vi "Test Assetion Results Records Assertion Type.vi"(8 "error in (no error)":errorcluster, 11 "Test Case In":refnum<class "Result Collector Tests.lvclass">) -> (0 "error out":errorcluster, 3 "Test Case Out":refnum<class "Result Collector Tests.lvclass">)   [LabVIEW 2020, in "Result Collector Tests.lvclass"]
uses:
  Result Collector Tests.lvclass
  C:/Program Files (x86)/National Instruments/LabVIEW 2020/vi.lib/Astemes/LUnit/Test Case.lvclass
  source/Framework/Result Collector/Result Collector.lvclass
  source/Rewrite Project/Result/Result.ctl
  source/Rewrite Project/Result/Status.ctl
  source/Rewrite Project/Result/Type.ctl
  source/Framework/Result Types/Assertion Result/Public/TypeDefs/Assertion Type.ctl
  source/Framework/Result Collector/Result Collector.lvclass/Result Collector.ctl
  <vilib>/Astemes/LUnit/Test Case.lvclass/Test Case.ctl
  7d523b10-b8d1-4baa-9334-5865d033fd32.vi
  source/Framework/Result Collector/Public/API/Collect Method Results.vi
  <vilib>/AdvancedString/Delimited String to 1D String Array.vi
  <vilib>/AdvancedString/1D String Array to Delimited String.vi
  source/Framework/Result Collector/Public/API/Collect Case Result.vi
  source/Framework/Result Collector/Public/API/Collect Suite Result.vi
  <vilib>/Astemes/LUnit/Palette/Pass.vi
  <vilib>/Astemes/LUnit/Palette/Fail.vi
  <vilib>/Astemes/LUnit/Compare Variants.vi
  <vilib>/Astemes/LUnit/Describe Comparison.vi
  <vilib>/Astemes/LUnit/Set Assertion Type.vi
  <vilib>/Astemes/LUnit/Add test result.vi
  <vilib>/Astemes/LUnit/Variant to string.vi
  <vilib>/Astemes/LUnit/LUnit Record Assertion Result.vi
  <vilib>/Astemes/LUnit/LUnit Aggregate Assertion Results.vi
  <vilib>/Astemes/LUnit/Method Result/LUnit Merge Status.vi
  <vilib>/Astemes/LUnit/LUnit Concatenate result strings.vi
  <vilib>/Utility/Data Type/Get Type Information.vi
  <vilib>/Utility/LVClass/Get LV Class Name.vi
  source/Rewrite Project/Result/Result.lvlib
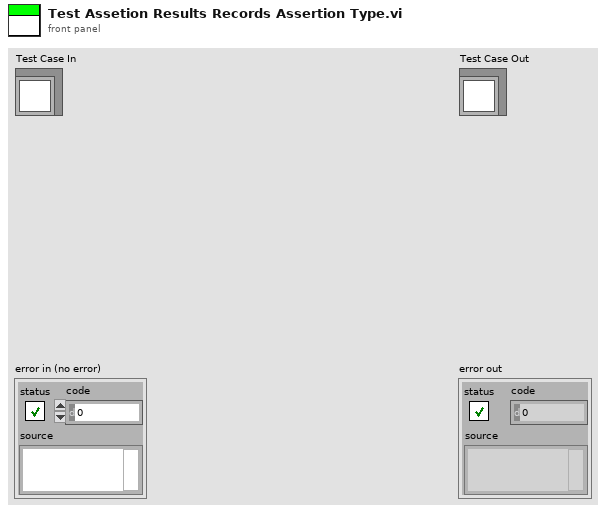
[diagram p1: front panel]
types:
  T1 = typedef "Result.lvlib/Assertion Type.ctl" = enum16{"None", "Pass", "Fail", "Skip", "Pass if Equal", "Fail if Equal", "Pass if Error", "Fail if Error", "Pass if", "Fail if"}
  T2 = typedef "Result.lvlib/Result.ctl" = cluster{"Name":string, "Message":string, "Description":string, "Status":T3, "Result Type":T4, "Execution Time":dbl}
  T3 = typedef "Result.lvlib/Status.ctl" = enum16{"", "Passed", "Failed", "Error", "Skipped", "Setup Error", "Broken", "Teardown Error"}
  T4 = typedef "Result.lvlib/Type.ctl" = enum16{"Method", "Case", "Suite", "Pass", "Fail", "Skip", "Pass if", "Fail if", "Pass if Error", "Fail if Error", "Pass if Equal", "Fail if Equal"}
  T5 = typedef "Assertion Result.lvlib/Assertion Result.ctl" = cluster{"Status":T3, "Message":string, "Description":string, "Assertion Type":T1}
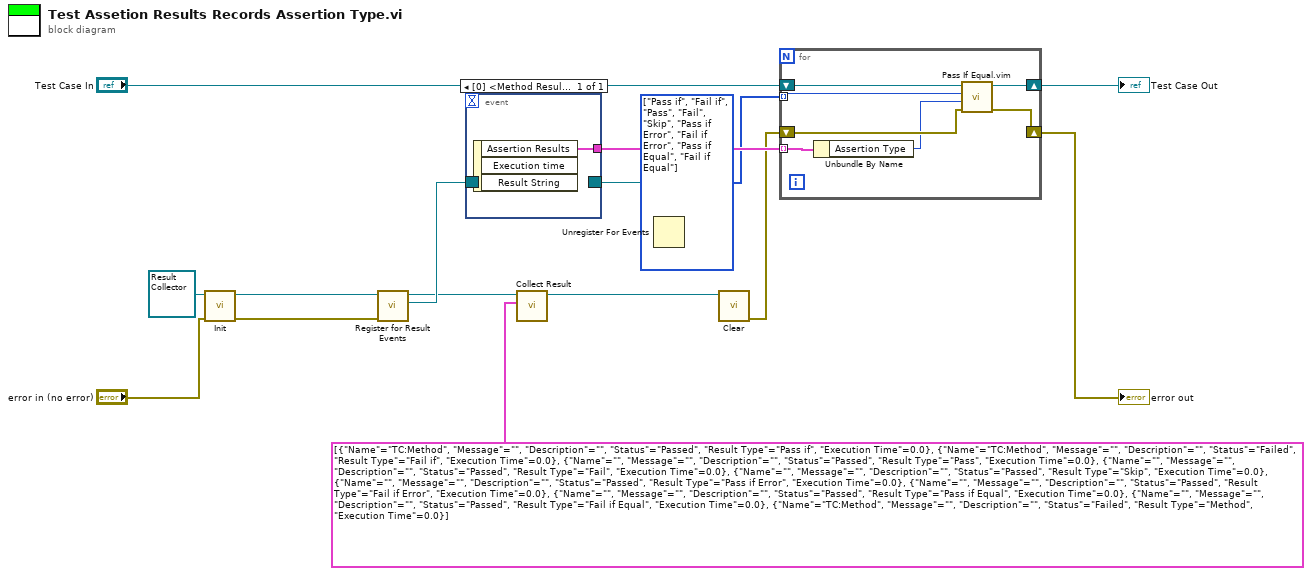
[diagram p0: block diagram]
diagram:
  w1 = T1[] [enum."Pass if", enum."Fail if", enum."Pass", enum."Fail", enum."Skip", enum."Pass if Error", enum."Fail if Error", enum."Pass if Equal", enum."Fail if Equal"] items=["None", "Pass", "Fail", "Skip", "Pass if Equal", "Fail if Equal", "Pass if Error", "Fail if Error", "Pass if", "Fail if"] ("Array")
  n1 = call-dynamic "Init.vi"("error in (no error)"="error in (no error)", "Report Generator In"=refnum<class "Result Collector.lvclass"> refnum) -> ("error out"=w11:errorcluster, "Report Generator Out"=w12:refnum<class "Result Collector.lvclass">)  [unwired: 8 in]
  n2 = call "Register for Result Events.vi"("error in (no error)"=w11, "Result Collector In"=w12) -> ("Event Registration Refnum"=w9:refnum<event-registration>, "Result Collector Out"=w7:refnum<class "Result Collector.lvclass">)  [unwired: 7 in, 1 out]
  n3 = event shown="[0] <Method Results>: User Event" {
    selector: w9 -> [_]
    dyn-events: [_] -> w8
    timeout: _ -> [_]
    tunnel: [w16] -> w4
    event User Event {
      n4 = event-data() -> ("Assertion Results"=w16:T5[])  [unwired: 1 in, 2 out]
    }
  }
  n5 = call "Collect Result.vi"("Results"=T2[] [{"Name"="TC:Method", "Message"="", "Description"="", "Status"=enum."Passed", "Result Type"=enum."Pass if", "Execution Time"=0.0}, {"Name"="TC:Method", "Message"="", "Description"="", "Status"=enum."Failed", "Result Type"=enum."Fail if", "Execution Time"=0.0}, {"Name"="", "Message"="", "Description"="", "Status"=enum."Passed", "Result Type"=enum."Pass", "Execution Time"=0.0}, {"Name"="", "Message"="", "Description"="", "Status"=enum."Passed", "Result Type"=enum."Fail", "Execution Time"=0.0}, {"Name"="", "Message"="", "Description"="", "Status"=enum."Passed", "Result Type"=enum."Skip", "Execution Time"=0.0}, {"Name"="", "Message"="", "Description"="", "Status"=enum."Passed", "Result Type"=enum."Pass if Error", "Execution Time"=0.0}, {"Name"="", "Message"="", "Description"="", "Status"=enum."Passed", "Result Type"=enum."Fail if Error", "Execution Time"=0.0}, {"Name"="", "Message"="", "Description"="", "Status"=enum."Passed", "Result Type"=enum."Pass if Equal", "Execution Time"=0.0}, {"Name"="", "Message"="", "Description"="", "Status"=enum."Passed", "Result Type"=enum."Fail if Equal", "Execution Time"=0.0}, {"Name"="TC:Method", "Message"="", "Description"="", "Status"=enum."Failed", "Result Type"=enum."Method", "Execution Time"=0.0}], "Report Generator In"=w7) -> ("Report Generator Out"=w6:refnum<class "Result Collector.lvclass">)  [unwired: 9 in]
  n6 = Unregister For Events(event registration refnum=w8) -> ()  [unwired: 1 in, 1 out]
  n7 = call-dynamic "Clear.vi"("Report Generator In"=w6) -> ("error out"=w3:errorcluster)  [unwired: 9 in, 1 out]
  n8 = for {
    tunnel: w4 -> [w21] mode=indexing
    shift-right: [w23] -> w14
    shift-left: "Test Case In" -> [w20]
    shift-right: [w22] -> w13
    shift-left: w3 -> [w19]
    tunnel: w1 -> [w18] mode=indexing
    n9 = Unbundle By Name(w21) -> ("Assertion Type"=w17:T1)
    n10 = call "Pass If Equal.vim"("error in (no error)"=w19, "Actual"=w17, "Expected"=w18, "LUnit Test Case In"=w20) -> ("error out"=w22:errorcluster, "LUnit Test Case Out"=w23:refnum<class "Result Collector Tests.lvclass">)  [unwired: 6 in]
  }
  "error out" <- w13
  "Test Case Out" <- w14
